vi "4 probe data-osc-time v1.8.vi"() -> ()   [LabVIEW 2014]
uses:
  <instrlib>/Tektronix TDS 200 1000 2000 Series/Tektronix TDS 200 1000 2000 Series.lvlib
panel:
  out "Waveform Data 2":waveform(dbl)(graph)
  out "Data IV Keithley 4":string
  in  "Data IV Keithley 3":path=path "c:/myfile.txt"
  out "Waveform Data":waveform(dbl)(graph)
  out "Seconds":sgl
  in  "stop button":bool
  in  "loop num":dbl=10000000000.0
  out "Data IV Keithley":string
  in  "Data IV Keithley 2":path=path "c:/myfile.txt"
  in  "Stop Button":bool
  in  "Channel 2 (1: Channel 2)":u16(ring)=1 items=["Channel 1", "Channel 2", "Channel 3", "Channel 4", "Math", "Reference A", "Reference B", "Reference C", "Reference D"]
  in  "Channel 1 (0: Channel 1)":u16(ring) items=["Channel 1", "Channel 2", "Channel 3", "Channel 4", "Math", "Reference A", "Reference B", "Reference C", "Reference D"]
  in  "Serial Configuration":T1={"Baud Rate"=9600, "Parity"=0, "Stop Bits"=10, "Flow Control"=2} {"Flow Control" items=["None", "XON/XOFF", "RTS/CTS", "XON/XOFF & RTS/CTS", "DTR/DSR", "XON/XOFF & DTR/DSR"]; "Stop Bits" items=["1.0"=10, "1.5"=15, "2.0"=20]; "Parity" items=["None", "Odd", "Even", "Mark", "Space"]; "Baud Rate" items=["300"=300, "600"=600, "1200"=1200, "2400"=2400, "4800"=4800, "9600"=9600, "19200"=19200]}
  in  "Probe Attenuation 2 (0.1)":dbl=0.1
  in  "Vertical Coupling 2 (1: DC)":u16(ring)=1 items=["AC", "DC", "Ground"]
  in  "Probe Attenuation 1 (0.1)":dbl=0.1
  in  "Vertical Coupling 1 (1: DC)":u16(ring)=1 items=["AC", "DC", "Ground"]
  in  "Timeout (10000 ms)":u32=500
  in  "VISA resource name":refnum<visa-resource-name>="USB0::0x0699::0x03A6::C044157::INSTR"
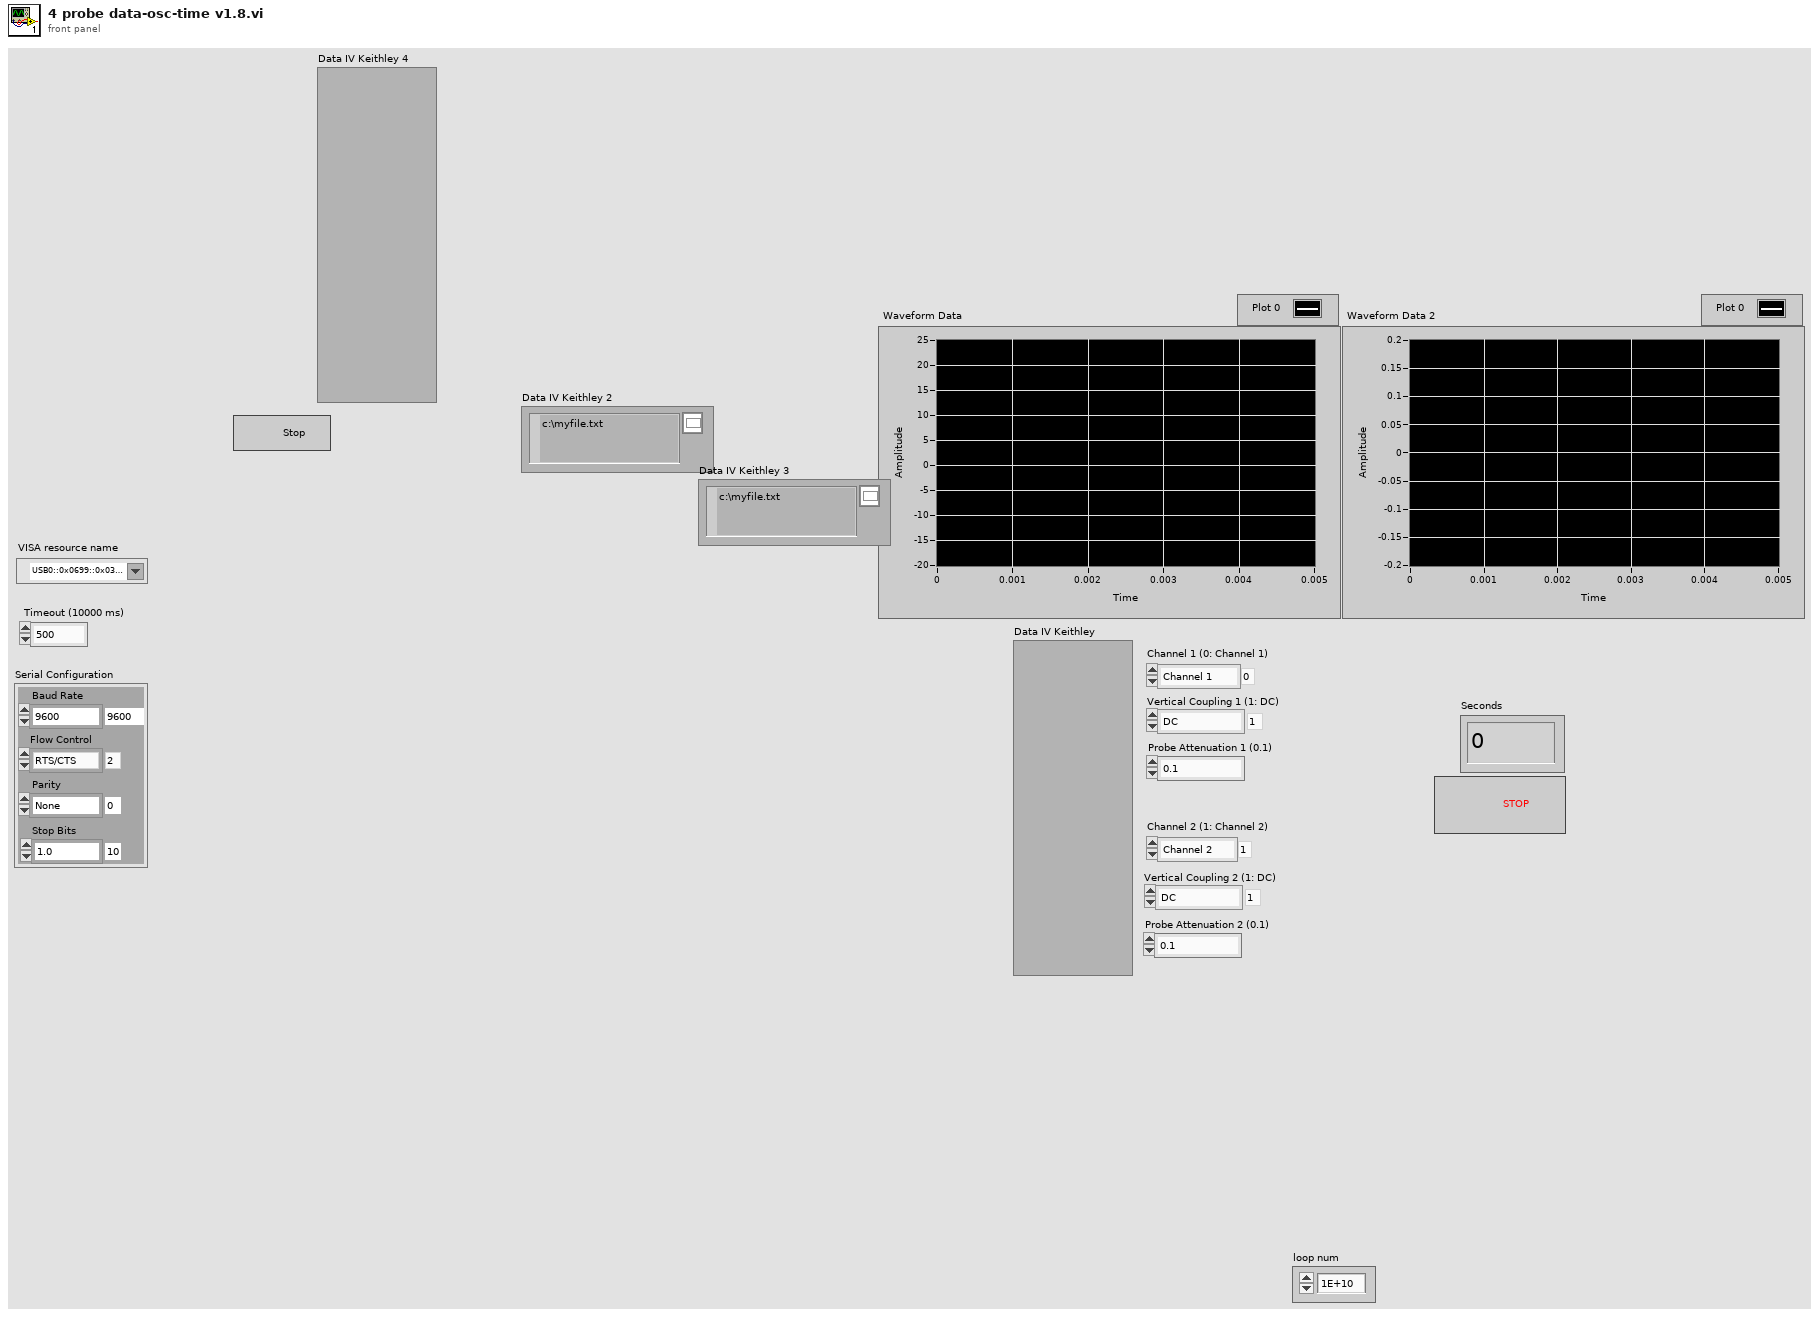
[diagram p1: front panel]
types:
  T1 = cluster{"Baud Rate":u32, "Parity":u16, "Stop Bits":u16, "Flow Control":u16}
  T2 = enum16{"open", "replace", "create", "open or create", "replace or create", "replace or create with confirmation"}
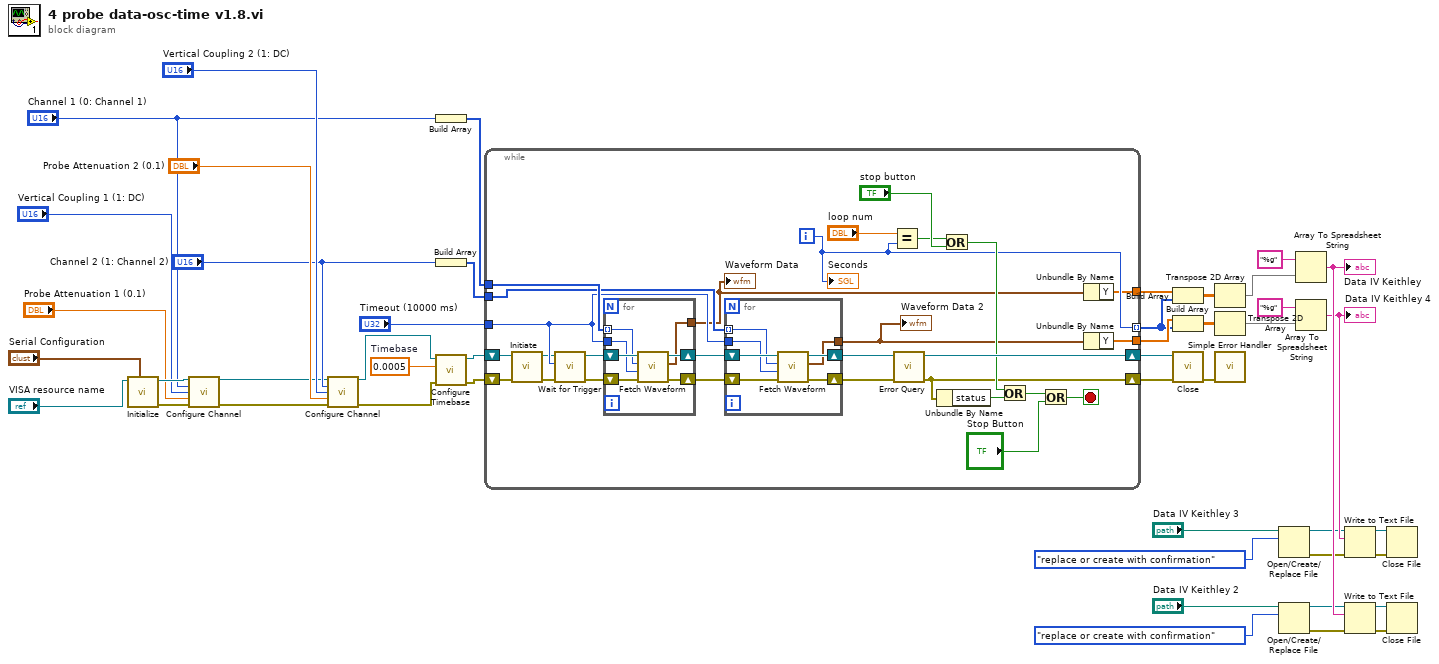
[diagram p0: block diagram]
diagram:
  w32 = 0.0005  # Timebase
  n1 = call <instrlib>:"Initialize.vi"("Serial Configuration"="Serial Configuration", "VISA resource name"="VISA resource name") -> ("error out"=w41:errorcluster, "VISA resource name out"=w42:refnum<visa-resource-name>)  [unwired: 3 in, 5 out]
  n2 = call <instrlib>:"Configure Channel.vi"("VISA resource name"=w42, "Channel (0: Channel 1)"="Channel 1 (0: Channel 1)", "Vertical Coupling (1: DC)"="Vertical Coupling 1 (1: DC)", "Probe Attenuation (10: 10X)"="Probe Attenuation 1 (0.1)", "error in (no error)"=w41) -> ("VISA resource name out"=w2:refnum<visa-resource-name>, "error out"=w1:errorcluster)  [unwired: 4 in, 5 out]
  n3 = call <instrlib>:"Configure Channel.vi"("VISA resource name"=w2, "Channel (0: Channel 1)"="Channel 2 (1: Channel 2)", "Vertical Coupling (1: DC)"="Vertical Coupling 2 (1: DC)", "Probe Attenuation (10: 10X)"="Probe Attenuation 2 (0.1)", "error in (no error)"=w1) -> ("VISA resource name out"=w40:refnum<visa-resource-name>, "error out"=w39:errorcluster)  [unwired: 4 in, 5 out]
  n4 = Build Array("Channel 1 (0: Channel 1)") -> (w31:u16[])
  n5 = Build Array("Channel 2 (1: Channel 2)") -> (w26:u16[])
  n6 = call <instrlib>:"Configure Timebase.vi"("error in (no error)"=w39, "Timebase (0.0005 s)"=w32, "VISA resource name"=w40) -> ("error out"=w37:errorcluster, "VISA resource name out"=w38:refnum<visa-resource-name>)  [unwired: 1 in, 6 out]
  n7 = while {
    tunnel: w31 -> [w71]
    tunnel: "Timeout (10000 ms)" -> [w70]
    tunnel: w26 -> [w69]
    shift-right: [w74] -> w44
    shift-left: w38 -> [w73]
    shift-right: [w57] -> w43
    shift-left: w37 -> [w72]
    tunnel: [w53] -> w3 mode=indexing
    tunnel: [w50] -> w15
    tunnel: [w48] -> w4
    i -> [w53]
    stop <- w54 stop-if-true
    n8 = call <instrlib>:"Initiate.vi"("error in (no error)"=w72, "VISA resource name"=w73) -> ("error out"=w65:errorcluster, "VISA resource name out"=w68:refnum<visa-resource-name>)  [unwired: 8 out]
    n9 = call <instrlib>:"Wait for Trigger.vi"("error in (no error)"=w65, "Timeout (10000 ms)"=w70, "VISA resource name"=w68) -> ("error out"=w66:errorcluster, "VISA resource name out"=w67:refnum<visa-resource-name>)  [unwired: 7 out]
    n10 = for {
      shift-right: [w87] -> w63
      shift-left: w66 -> [w85]
      tunnel: w71 -> [w83] mode=indexing
      tunnel: w70 -> [w84]
      shift-right: [w88] -> w64
      shift-left: w67 -> [w86]
      tunnel: [w82] -> w49
      n11 = call <instrlib>:"Fetch Waveform.vi"("error in (no error)"=w85, "Timeout (10000 ms)"=w84, "Source (0: Channel 1)"=w83, "VISA resource name"=w86) -> ("error out"=w87:errorcluster, "Waveform Data"=w82:waveform(dbl), "VISA resource name out"=w88:refnum<visa-resource-name>)  [unwired: 2 in, 3 out]
    }
    "Waveform Data" <- w49
    n12 = for {
      shift-right: [w80] -> w51
      shift-left: w63 -> [w78]
      tunnel: w69 -> [w76] mode=indexing
      tunnel: w70 -> [w77]
      shift-right: [w81] -> w52
      shift-left: w64 -> [w79]
      tunnel: [w75] -> w47
      n13 = call <instrlib>:"Fetch Waveform.vi"("error in (no error)"=w78, "Timeout (10000 ms)"=w77, "Source (0: Channel 1)"=w76, "VISA resource name"=w79) -> ("error out"=w80:errorcluster, "Waveform Data"=w75:waveform(dbl), "VISA resource name out"=w81:refnum<visa-resource-name>)  [unwired: 2 in, 3 out]
    }
    "Waveform Data 2" <- w47
    n14 = Equal?(x="loop num", y=w53) -> (x = y?=w58:bool)
    n15 = call <instrlib>:"Error Query.vi"("error in (no error)"=w51, "VISA resource name"=w52) -> ("error out"=w57:errorcluster, "VISA resource name out"=w74:refnum<visa-resource-name>)  [unwired: 8 out]
    n16 = Unbundle By Name(w57) -> ("status"=w60:bool)
    n17 = Or(x=w58, y="stop button") -> (x .or. y?=w59:bool)
    n18 = Or(x=w59, y=w60) -> (x .or. y?=w56:bool)
    n19 = Or(x=w56, y="Stop Button") -> (x .or. y?=w54:bool)
    n20 = Unbundle By Name(w49) -> ("Y"=w50:dbl[])
    n21 = Unbundle By Name(w47) -> ("Y"=w48:dbl[])
    "Seconds" <- w53
  }
  n22 = Build Array(w15, w3) -> (w22:dbl[][])
  n23 = Build Array(w4, w3) -> (w11:dbl[][])
  n24 = call <instrlib>:"Close.vi"("error in (no error)"=w43, "VISA resource name"=w44) -> ("error out"=w45:errorcluster)  [unwired: 9 out]
  n25 = Transpose 2D Array(2D array=w22) -> (transposed array=w24:dbl[][])
  n26 = Transpose 2D Array(2D array=w11) -> (transposed array=w13:dbl[][])
  n27 = call <vilib>:"Simple Error Handler.vi"("error in (no error)"=w45) -> ()  [unwired: 1 in, 8 out]
  n28 = Open/Create/Replace File(file path (use dialog)="Data IV Keithley 3", operation (0:open)=T2."replace or create with confirmation") -> (refnum out=w10:refnum<file>, error out=w5:errorcluster)  [unwired: 4 in, 1 out]
  n29 = Open/Create/Replace File(file path (use dialog)="Data IV Keithley 2", operation (0:open)=T2."replace or create with confirmation") -> (refnum out=w21:refnum<file>, error out=w16:errorcluster)  [unwired: 4 in, 1 out]
  n30 = Array To Spreadsheet String(array=w24, 3:"%g" ("format string")) -> (spreadsheet string=w25:string)  [unwired: 1 in]
  "Data IV Keithley" <- w25
  n31 = Array To Spreadsheet String(array=w13, 3:"%g" ("format string")) -> (spreadsheet string=w14:string)  [unwired: 1 in]
  "Data IV Keithley 4" <- w14
  n32 = Write to Text File(file (use dialog)=w10, text=w14, error in=w5) -> (refnum out=w7:refnum<file>, error out=w6:errorcluster)  [unwired: 2 out]
  n33 = Write to Text File(file (use dialog)=w21, text=w25, error in=w16) -> (refnum out=w18:refnum<file>, error out=w17:errorcluster)  [unwired: 2 out]
  n34 = Close File(refnum=w7, error in=w6) -> ()  [unwired: 2 out]
  n35 = Close File(refnum=w18, error in=w17) -> ()  [unwired: 2 out]
